vi "Configure Channel.vi"(0 "VISA resource name":refnum<visa-resource-name>, 1 "Enable Channel (T:On)":bool=TRUE, 2 "Bandwidth (0: Full)":u16(ring) items=["Full", "20MHZ", "25MHZ", "200MHZ", "250MHZ", "1GHZ", "3GHZ", "4GHZ"], 5 "Channel (0: Channel 1)":u16(ring) items=["Channel 1", "Channel 2", "Channel 3", "Channel 4"], 7 "Vertical Coupling (0: A1M)":u16(ring) items=["A1M", "D1M", "D50", "Ground", "DC", "AC"], 9 "Probe Attenuation (-1.0)":dbl=-1.0, 11 "error in (no error)":errorcluster, 12 "Vertical Range (10.0 V)":dbl=10.0, 13 "Vertical Offset (0.0 V)":dbl) -> (4 "VISA resource name out":refnum<visa-resource-name>, 15 "error out":errorcluster)   [LabVIEW 2018, in "LeCroy Wave Series.lvlib"]
doc: "Configures the common properties of the oscilloscope's vertical subsystem for the specified channel. Call this VI for each channel you want to enable to acquire waveforms.\n\nCaveats:\n1. The oscilloscope will not accept a value for Probe Attenuation if there is a probe attached that employs a fixed value for attenuation.\n2. Allowed coupling values depend on what kind of probe is attached, if any.\n\nNote:\nThe channel settings will not be applied if the channel is not enabled."
uses:
  LeCroy Wave Series.lvlib
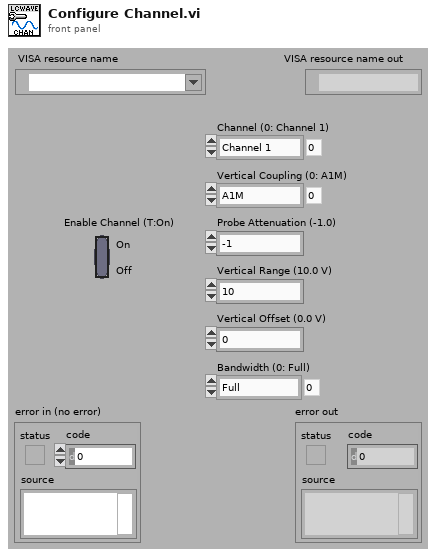
[diagram p1: front panel]
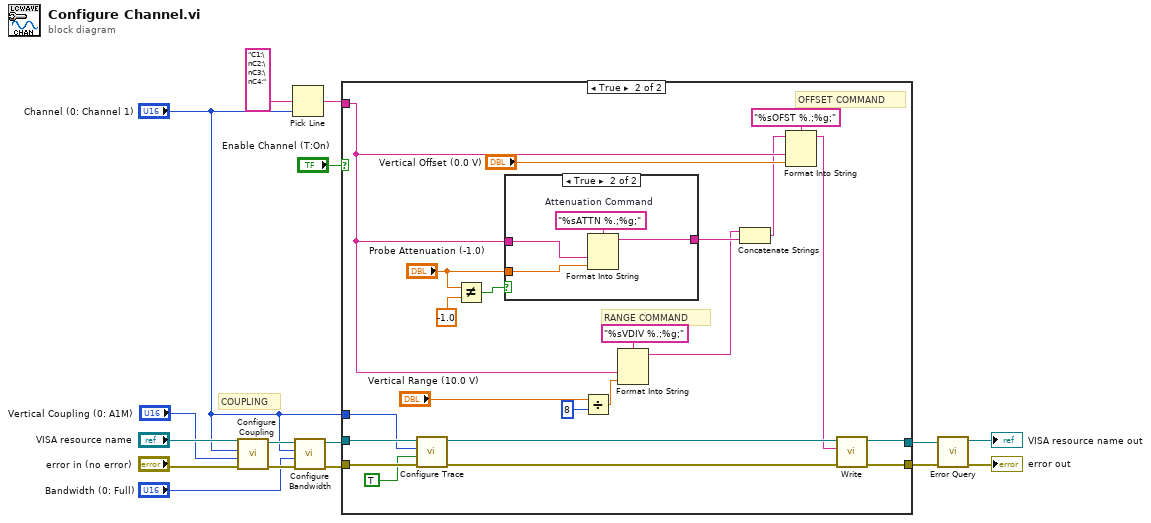
[diagram p0: block diagram]
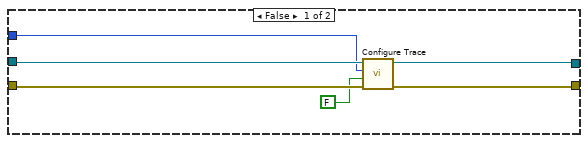
[diagram p2: hidden frame]
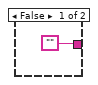
[diagram p3: hidden frame]
diagram:
  # "COUPLING"
  n1 = call "Configure Coupling.vi"("error in (no error)"="error in (no error)", "Vertical Coupling (0: A1M)"="Vertical Coupling (0: A1M)", "Channel (0: Channel 1)"="Channel (0: Channel 1)", "VISA resource name"="VISA resource name") -> ("error out"=w9:errorcluster, "VISA resource name out"=w10:refnum<visa-resource-name>)  [unwired: 6 in]
  n2 = Pick Line(multi-line string="C1:\nC2:\nC3:\nC4:", line index="Channel (0: Channel 1)") -> (output string=w14:string)  [unwired: 1 in]
  n3 = call "Configure Bandwidth.vi"("error in (no error)"=w9, "Bandwidth Limit (0: Full)"="Bandwidth (0: Full)", "Channel (0: Channel 1)"="Channel (0: Channel 1)", "VISA resource name"=w10) -> ("error out"=w8:errorcluster, "VISA resource name out"=w7:refnum<visa-resource-name>)  [unwired: 6 in]
  n4 = case shown="True" "Enable Channel (T:On)" {
    tunnel: w14 -> [_ w32]
    tunnel: w7 -> [w22 w36]
    tunnel: w8 -> [w21 w35]
    tunnel: [w19 w38] -> w2
    tunnel: [w20 w37] -> w1
    tunnel: "Channel (0: Channel 1)" -> [w18 w33]
    frame False {
      n5 = call "Configure Trace.vi"("error in (no error)"=w21, "Enable Trace Mode (T: Enable)"=FALSE ("Mode"), "Trace (0: Channel 1)"=w18, "VISA resource name"=w22) -> ("error out"=w20:errorcluster, "VISA resource name out"=w19:refnum<visa-resource-name>)  [unwired: 6 in]
    }
    frame True {
      # "RANGE COMMAND"
      # "OFFSET COMMAND"
      n6 = call "Configure Trace.vi"("error in (no error)"=w35, "Enable Trace Mode (T: Enable)"=TRUE ("Mode"), "Trace (0: Channel 1)"=w33, "VISA resource name"=w36) -> ("error out"=w26:errorcluster, "VISA resource name out"=w27:refnum<visa-resource-name>)  [unwired: 6 in]
      n7 = Not Equal?(x="Probe Attenuation (-1.0)", y=-1.0 ("x")) -> (x != y?=w41:bool)
      n8 = case shown="True" w41 {
        tunnel: w32 -> [_ w48]
        tunnel: "Probe Attenuation (-1.0)" -> [_ w47]
        tunnel: ["" ("Empty String Constant") w46] -> w28
        frame False {
        }
        frame True {
          w49 = "%sATTN %.;%g;"  # Attenuation Command
          n9 = Format Into String(format string=w49, w48, w47) -> (resulting string=w46:string)  [unwired: 2 in, 1 out]
        }
      }
      n10 = Divide(x="Vertical Range (10.0 V)", y=8) -> (x/y=w31:dbl)
      n11 = Format Into String(format string="%sVDIV %.;%g;", w32, w31) -> (resulting string=w25:string)  [unwired: 2 in, 1 out]
      n12 = Concatenate Strings(w25, w28) -> (w24:string)
      n13 = Format Into String(format string="%sOFST %.;%g;", initial string=w24, w32, "Vertical Offset (0.0 V)") -> (resulting string=w23:string)  [unwired: 1 in, 1 out]
      n14 = call "Write.vi"("error in (no error)"=w26, "Write Buffer"=w23, "VISA resource name"=w27) -> ("error out"=w37:errorcluster, "VISA resource name out"=w38:refnum<visa-resource-name>)  [unwired: 7 in]
    }
  }
  n15 = call "Error Query.vi"("error in (no error)"=w1, "VISA resource name"=w2) -> ("error out"=→"error out":errorcluster, "VISA resource name out"=→"VISA resource name out":refnum<visa-resource-name>)  [unwired: 6 in, 2 out]
